vi "Main.vi"(8 "error in (no error)":errorcluster, 11 "CascadeBase in":refnum<class "Cascade.lvclass">) -> (0 "error out":errorcluster, 3 "component":refnum<class "Cascade.lvclass">)   [LabVIEW 2012, in "Cascade.lvclass"]
doc: "Main VI of the component."
uses:
  Cascade.lvclass
  <vilib>/Distrio/Murmex/Murmex/command_enum.ctl
  Cascade.lvclass/Cascade.ctl
  <vilib>/Distrio/Murmex/InitialiseMessage/InitialiseMessage.lvclass
  <vilib>/Distrio/Murmex/GenericMessage/GenericMessage.lvclass
  <vilib>/Distrio/Murmex/TerminateMessage/TerminateMessage.lvclass
  <vilib>/Distrio/Murmex/ConfigureMessage/ConfigureMessage.lvclass
  <vilib>/Distrio/Murmex/StartMessage/run mode enum.ctl
  <vilib>/Distrio/Murmex/StopMessage/StopMessage.lvclass
  <vilib>/Distrio/Murmex/StartMessage/StartMessage.lvclass
  <vilib>/Distrio/Murmex/Murmex/update_cluster.ctl
  <vilib>/Distrio/Murmex/Murmex/Murmex.lvclass
  <vilib>/Distrio/Murmex/Murmex/Set configure at initialise.vi
  <vilib>/Distrio/Murmex/Murmex/Set log reference.vi
  <vilib>/Distrio/Murmex/Murmex/Set VI reference.vi
  <vilib>/Distrio/Murmex/Murmex/Get ID.vi
  <vilib>/Distrio/Murmex/Murmex/Set write log to disk.vi
  <vilib>/Distrio/Murmex/Message/Add or replace parameter.vi
  <vilib>/Distrio/Murmex/Message/Message.lvclass
  <vilib>/vision/NI_Vision_Development_Module.lvlib
panel:
  in  "PID gains":T1
  in  "button:configure":bool
  in  "button:quit":bool
  out "terminate?":bool
  in  "Tab Control":enum32{"Settings", "Phase comparison", "Debug"}(tab)
  out "Video":T2(plugin-control)
  in  "Exposure":dbl[unit]
  in  "Gain":dbl=65535.0
  in  "button:free run":bool
  out "Status":string
  in  "Reporting folder":path=path "C:/DATA"
  in  "Filename":string="trial"
  in  "save":bool
  in  "select ROIS":bool
  out "good alignment?":bool
  out "translation":dbl[unit]
  out "pixel shift":dbl
  in  "send move":bool
  in  "AF":bool
  in  "set as focus":bool
  out "ROB":T2(plugin-control)
  out "rob":T2(plugin-control)
  out "ROY":T2(plugin-control)
  out "roy":T2(plugin-control)
  out "aligned ROIs":T2(plugin-control)
  out "log":string
  in  "Component id":string="Cascade"
  in  "button:send command":bool
  in  "generic command":string
  in  "command":T3
  in  "button:single frame":bool
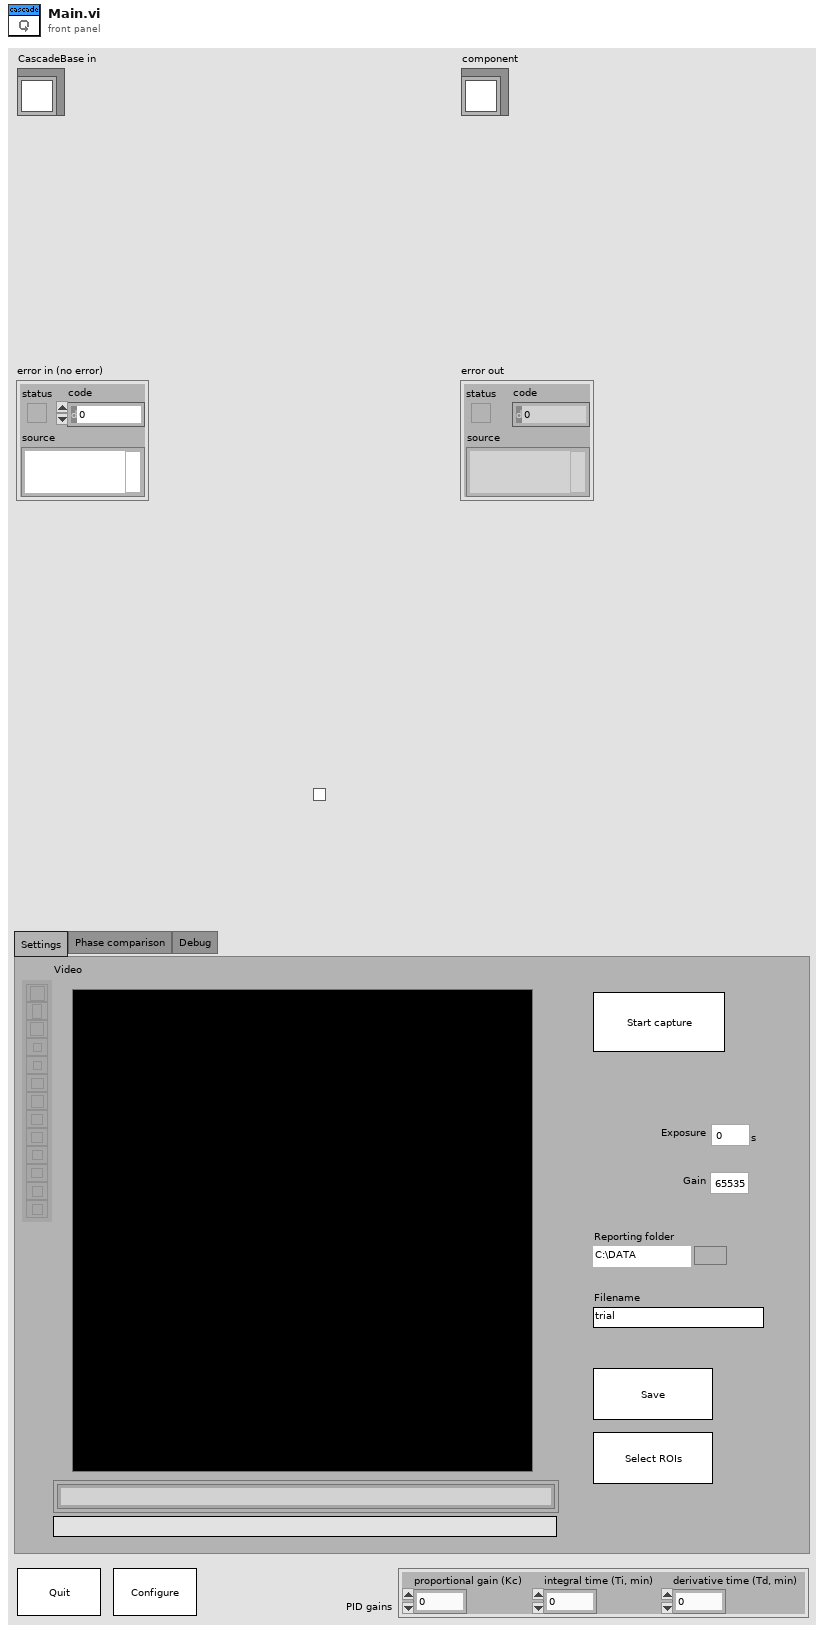
[diagram p1: front panel]
types:
  T1 = cluster{"proportional gain (Kc)":dbl, "integral time (Ti, min)":dbl, "derivative time (Td, min)":dbl}
  T2 = typedef "IMAQ Image.ctl" = refnum<image>
  T3 = typedef "Murmex.lvlib/Murmex.lvclass/command_enum.ctl" = enum16{"null", "initialise", "reset", "terminate", "acknowledge", "update", "inspect", "inform", "proceed", "start", "stop", "fetch", "configure", "generic"}
  T4 = enum8{"Enabled", "Disabled", "Disabled and Grayed Out"}
  T5 = typedef "Murmex.lvlib/StartMessage.lvclass/run mode enum.ctl" = enum16{"infinite", "finite"}
  T6 = typedef "Murmex.lvlib/Murmex.lvclass/update_cluster.ctl" = cluster{"target ID":string, "key chains":string[], "values":variant[]}
  T7 = typedef "Murmex.lvclass/command_enum.ctl" = enum16{"null", "initialise", "reset", "terminate", "acknowledge", "update", "inspect", "inform", "proceed", "start", "stop", "fetch", "configure", "generic"}
  T8 = typedef "Murmex.lvclass/Event type enumerations.ctl" = enum16{"before", "after"}
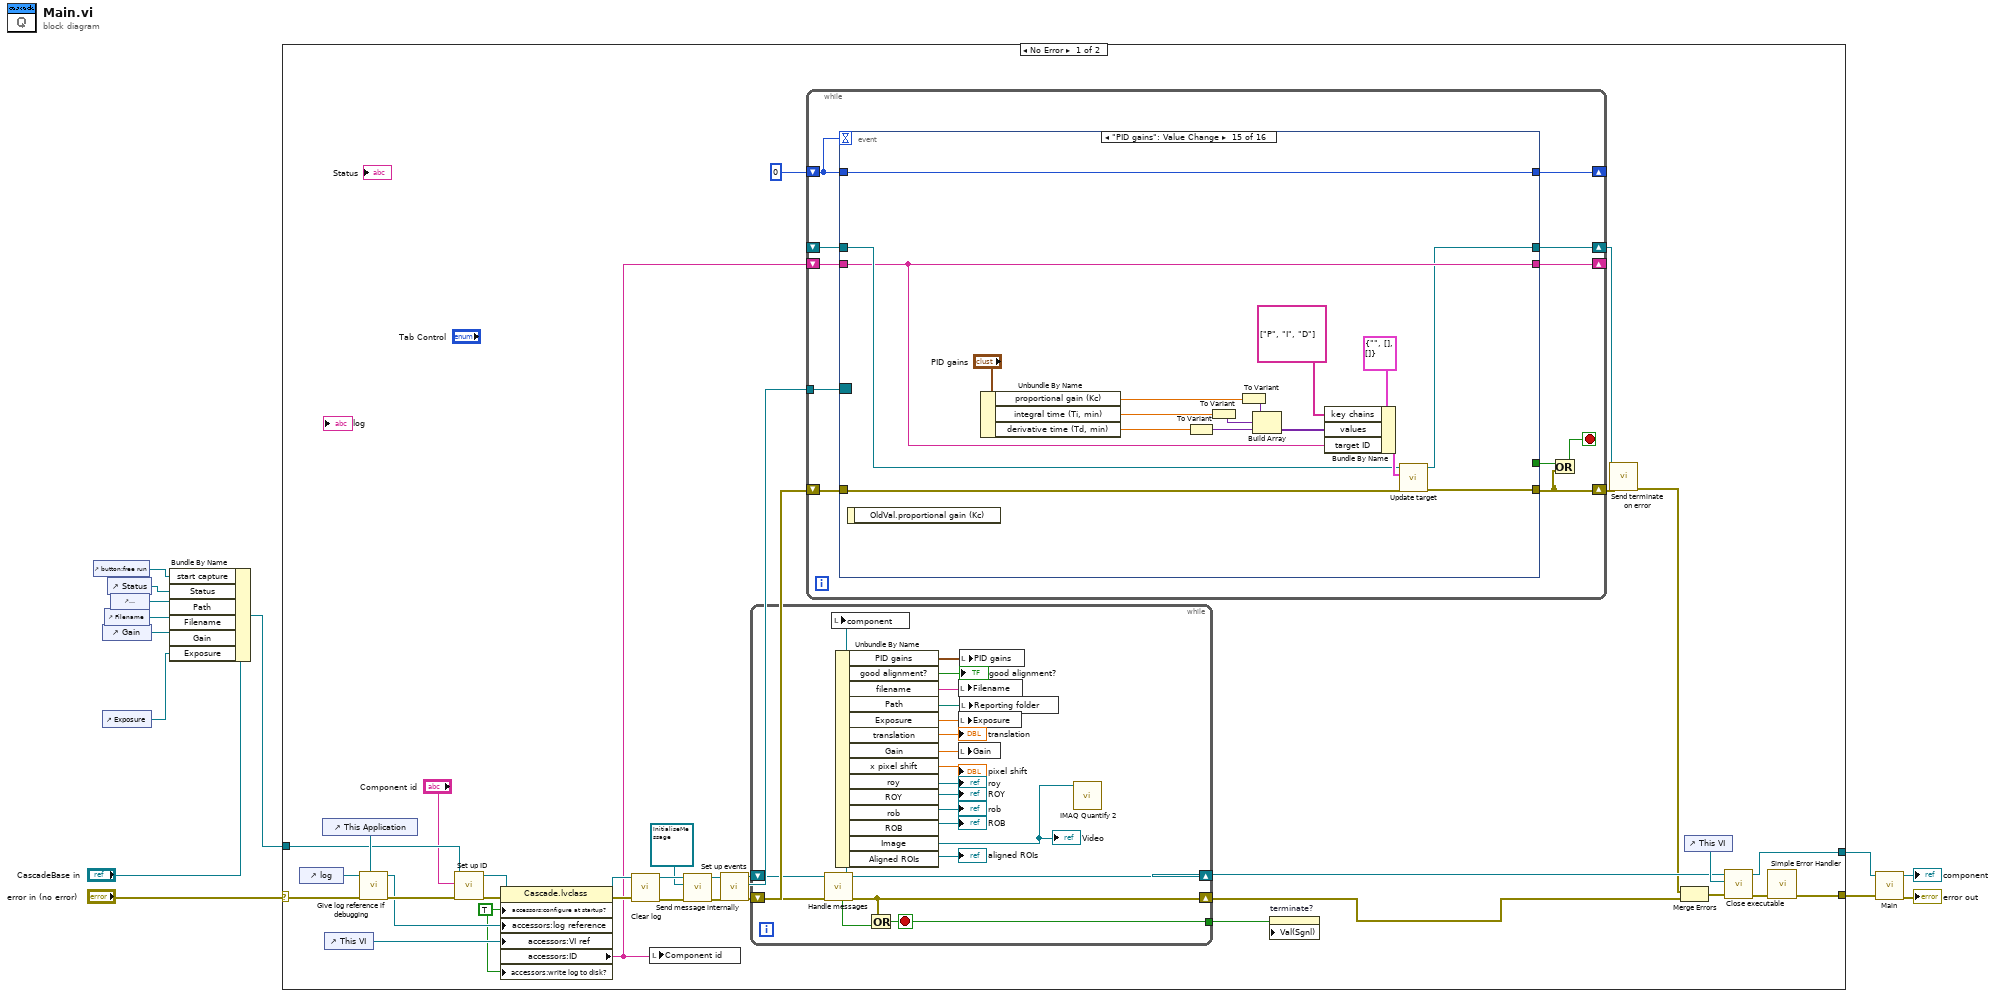
[diagram p0: block diagram]
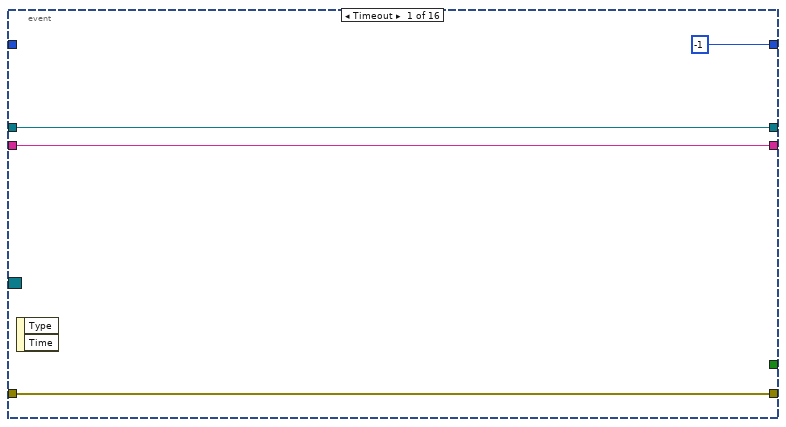
[diagram p2: hidden frame]
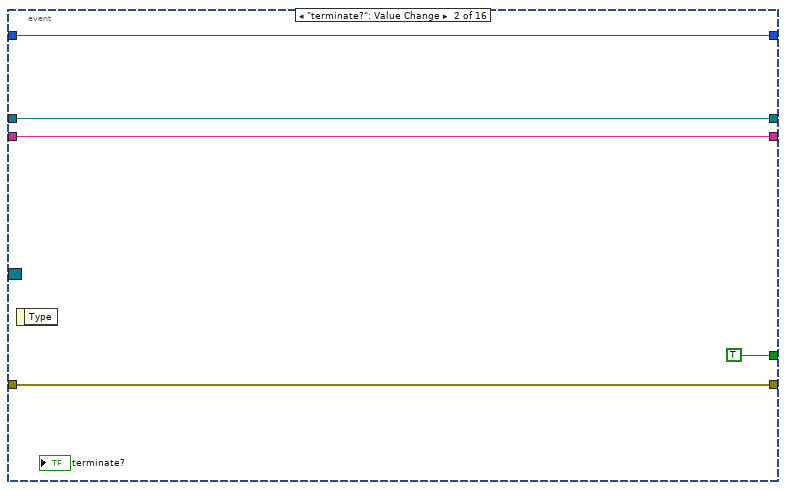
[diagram p3: hidden frame]
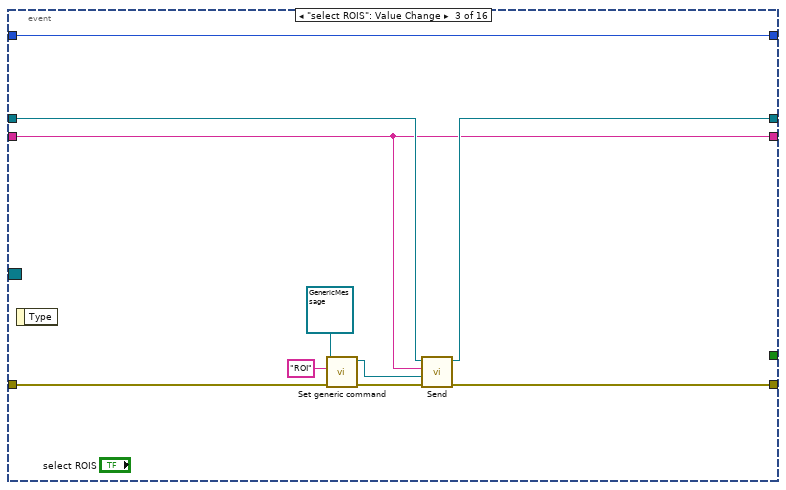
[diagram p4: hidden frame]
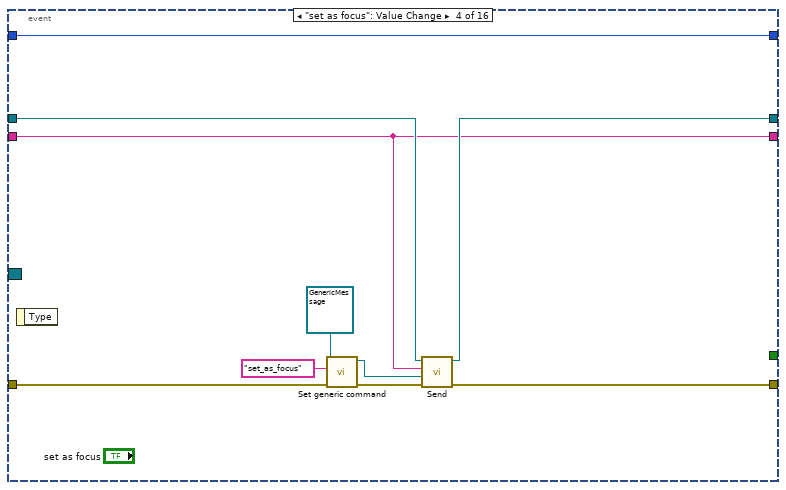
[diagram p5: hidden frame]
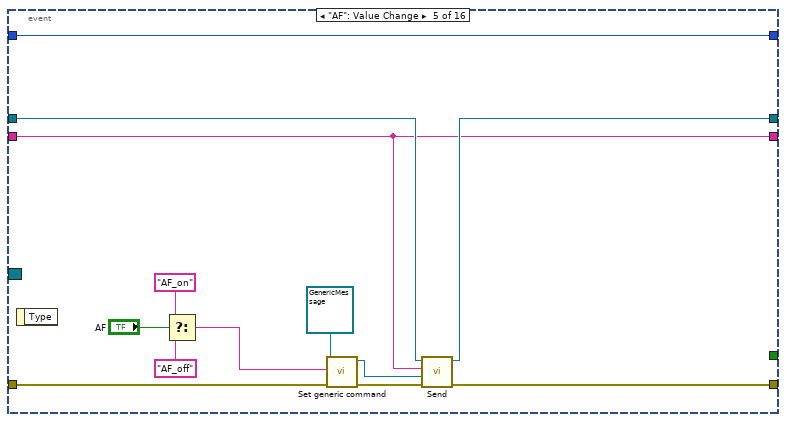
[diagram p6: hidden frame]
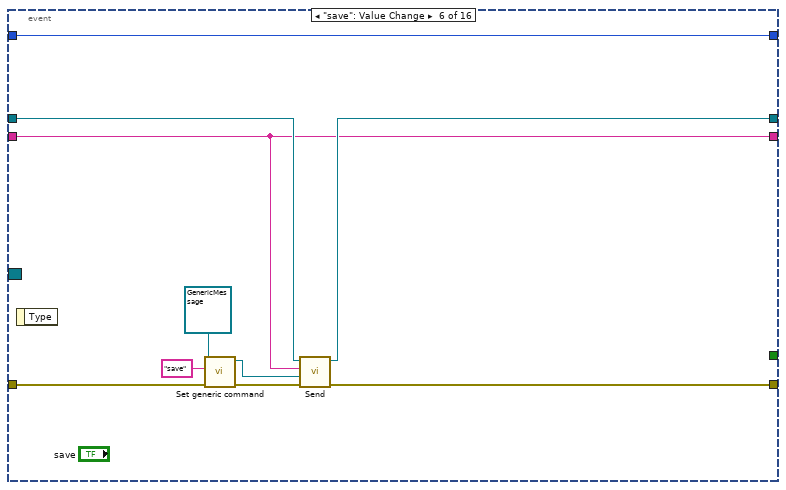
[diagram p7: hidden frame]
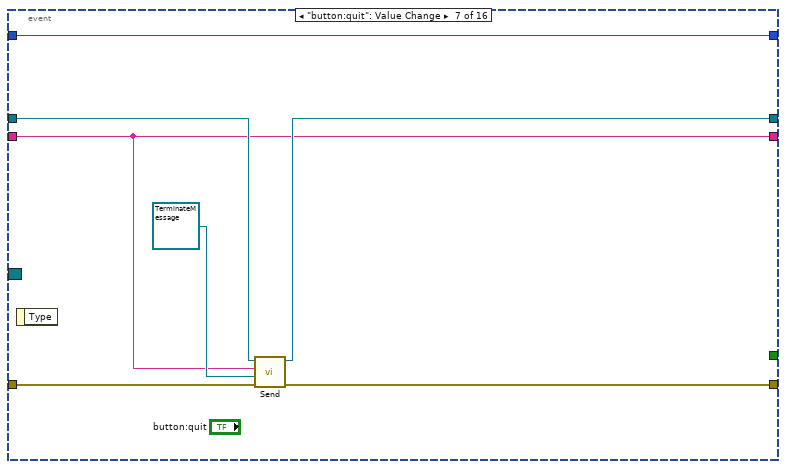
[diagram p8: hidden frame]
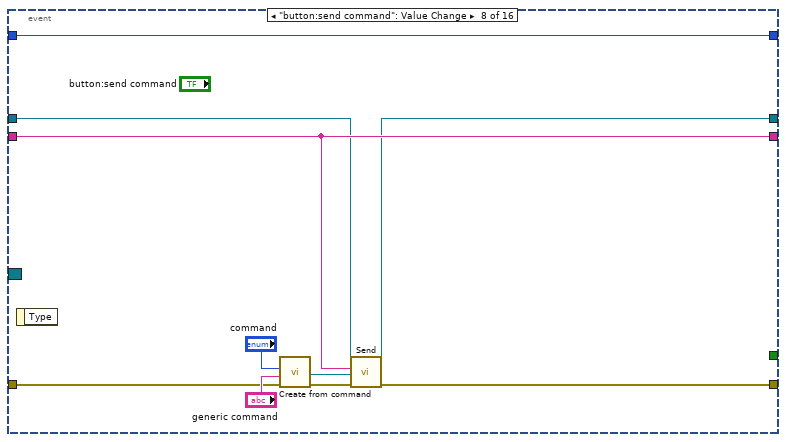
[diagram p9: hidden frame]
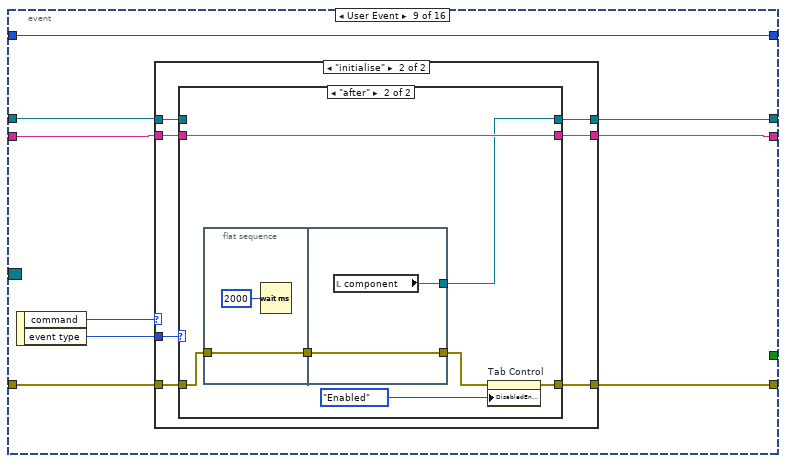
[diagram p10: hidden frame]
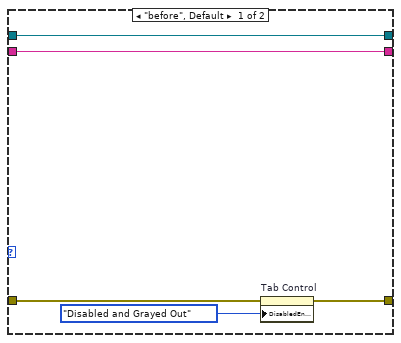
[diagram p12: hidden frame]
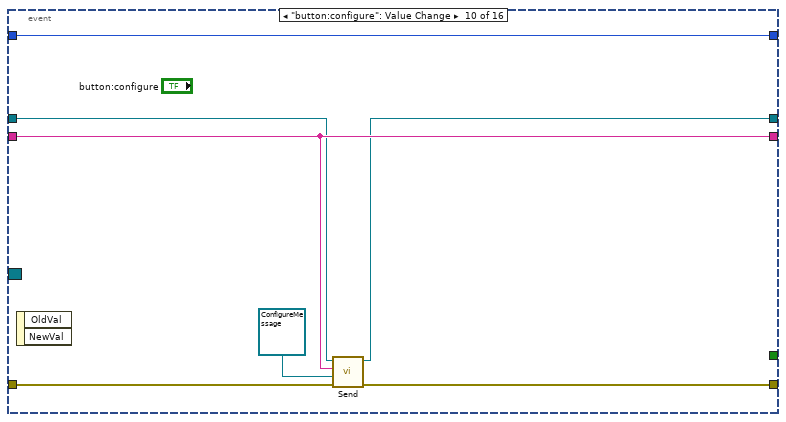
[diagram p13: hidden frame]
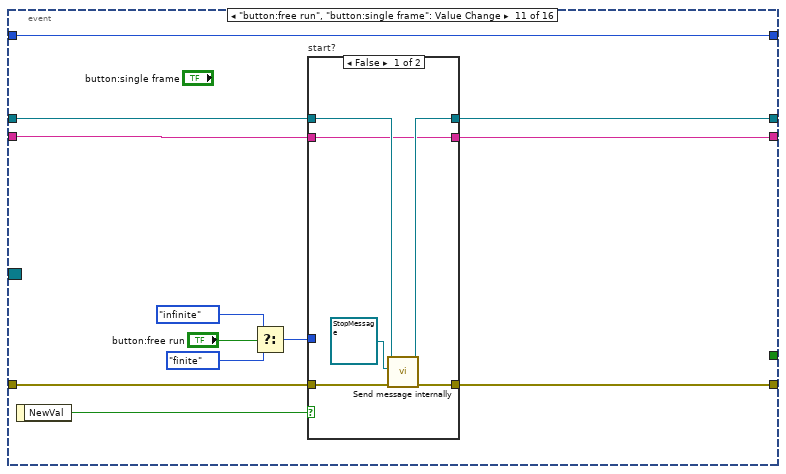
[diagram p14: hidden frame]
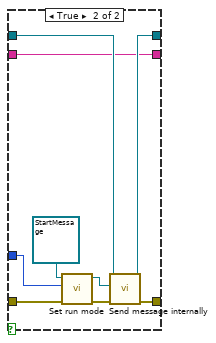
[diagram p15: hidden frame]
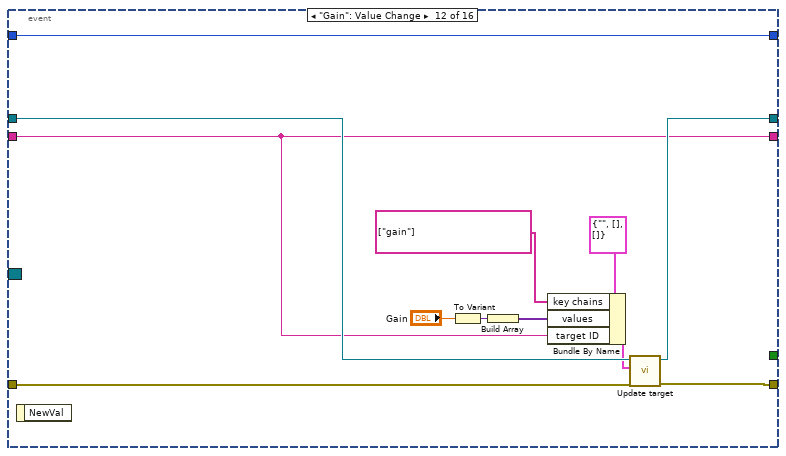
[diagram p16: hidden frame]
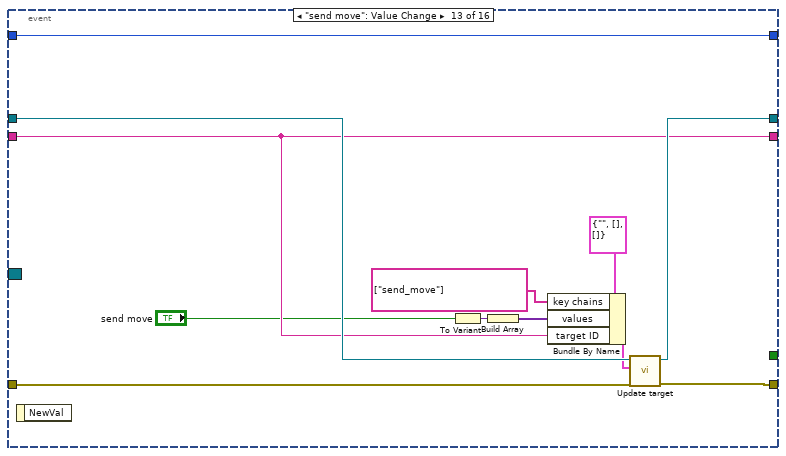
[diagram p17: hidden frame]
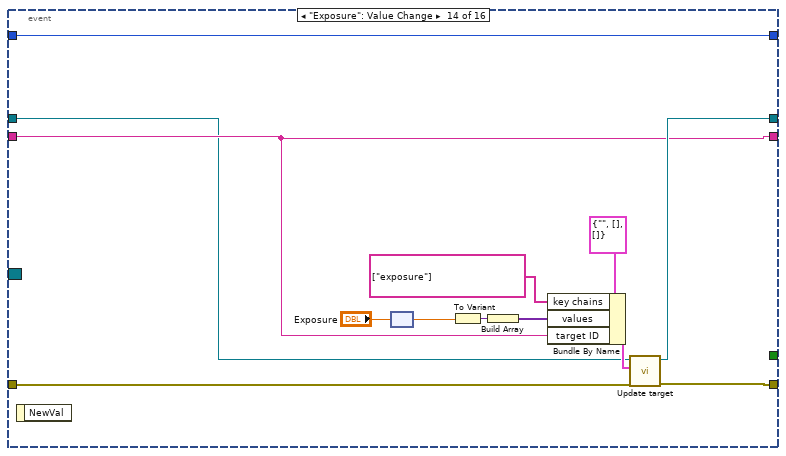
[diagram p18: hidden frame]
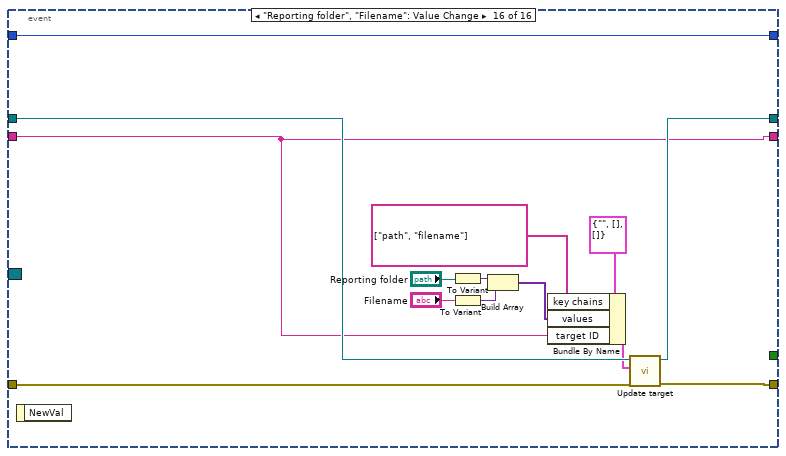
[diagram p19: hidden frame]
diagram:
  n1 = control-ref of="button:free run"() -> (w1:refnum<vi>)
  n2 = control-ref of="Gain"() -> (w5:refnum<vi>)
  n3 = control-ref of="Exposure"() -> (w6:refnum<vi>)
  n4 = control-ref of="Filename"() -> (w4:refnum<vi>)
  n5 = control-ref of="Status"() -> (w2:refnum<vi>)
  n6 = control-ref of="Reporting folder"() -> (w3:refnum<vi>)
  n7 = Bundle By Name(cluster="CascadeBase in", "start capture"=w1, "Status"=w2, "Path"=w3, "Filename"=w4, "Gain"=w5, "Exposure"=w6) -> (w10:refnum<class "Cascade.lvclass">)
  n8 = case shown="No Error" "error in (no error)" {
    selector: "error in (no error)" -> [w46 w286]
    tunnel: w10 -> [w45 w285]
    tunnel: [w19 w285] -> w9
    tunnel: [w17 w286] -> w7
    frame No Error {
      w15 = TRUE ("configure at startup?")
      n9 = control-ref of="log"() -> (w39:refnum<vi>)
      n10 = control-ref of="This Application"() -> (w47:refnum<vi>)
      n11 = control-ref of="This VI"() -> (w38:refnum<vi>)
      n12 = call "Give log reference if debugging.vi"("application ref"=w47, "error in (no error)"=w46, "log reference in"=w39) -> ("error out"=w44:errorcluster, "log reference out"=w40:refnum<vi>)  [unwired: 6 in, 1 out]
      n13 = call <vilib>:"Set up ID.vi"("error in (no error)"=w44, "component ID"="Component id", "MurmexBase in"=w45) -> ("error out"=w42:errorcluster, "MurmexBase out"=w41:refnum<class "Cascade.lvclass">)  [unwired: 6 in, 1 out]
      n14 = property class="Cascade.lvclass"(reference=w41, error in=w42, "accessors:configure at startup?"=w15, "accessors:log reference"=w40, "accessors:VI ref"=w38, "accessors:write log to disk?"=w15) -> (reference out=w31:refnum<class "Cascade.lvclass">, error out=w33:errorcluster, "accessors:ID"=w27:string)
      n15 = call <vilib>:"Clear log.vi"("error in (no error)"=w33, "MurmexBase in"=w31) -> ("error out"=w36:errorcluster, "MurmexBase out"=w37:refnum<class "Cascade.lvclass">)  [unwired: 8 in]
      n16 = local write "Component id"(w27) -> ()
      n17 = call <vilib>:"Send message internally.vi"("error in (no error)"=w36, "Message"=refnum<class "InitialiseMessage.lvclass"> refnum ("InitialiseMessage"), "Murmex in"=w37) -> ("error out"=w35:errorcluster, "Murmex out"=w34:refnum<class "Cascade.lvclass">)  [unwired: 7 in]
      n18 = call <vilib>:"Set up events.vi"("error in (no error)"=w35, "MurmexBase in"=w34) -> ("error out"=w28:errorcluster, "Event Registration Refnum"=w30:refnum<event-registration>, "MurmexBase out"=w29:refnum<class "Cascade.lvclass">)  [unwired: 7 in]
      n19 = while {
        shift-right: [w282] -> w14
        shift-left: w28 -> [w284]
        shift-right: [w279] -> w20
        shift-left: w29 -> [w280]
        tunnel: [w281] -> w16
        stop <- w281 stop-if-true
        n20 = call <vilib>:"Handle messages.vi"("error in (no error)"=w284, "Murmex in"=w280) -> ("error out"=w282:errorcluster, "Murmex out"=w279:refnum<class "Cascade.lvclass">, "terminated?"=w283:bool)  [unwired: 7 in]
        n21 = local write "component"(w279) -> ()
        n22 = Unbundle By Name(w279) -> ("PID gains"=w265:T1, "good alignment?"=→"good alignment?":bool, "filename"=w268:string, "Path"=w267:path, "Exposure"=w269:dbl[unit], "translation"=→"translation":dbl[unit], "Gain"=w270:dbl, "x pixel shift"=→"pixel shift":dbl, "roy"=→"roy":T2, "ROY"=→"ROY":T2, "rob"=→"rob":T2, "ROB"=→"ROB":T2, "Image"=w271:T2, "Aligned ROIs"=→"aligned ROIs":T2)
        "Video" <- w271
        n23 = Or(x=w282, y=w283) -> (x .or. y?=w281:bool)
        n24 = local write "Filename"(w268) -> ()
        n25 = local write "Exposure"(w269) -> ()
        n26 = local write "Gain"(w270) -> ()
        n27 = local write "PID gains"(w265) -> ()
        n28 = local write "Reporting folder"(w267) -> ()
        n29 = call "IMAQ Quantify 2"("Image"=w271) -> ()  [unwired: 8 in, 3 out]
      }
      n30 = while {
        tunnel: w30 -> [w58]
        shift-right: [w50] -> w25
        shift-left: w28 -> [w57]
        shift-right: [w55] -> _
        shift-left: 0 -> [w54]
        shift-right: [w53] -> _
        shift-left: w27 -> [w56]
        shift-right: [w52] -> w24
        shift-left: _ -> [w51]
        stop <- w49 stop-if-true
        n31 = event shown="[14] \"PID gains\": Value Change" {
          selector: w58 -> [_ _ _ _ _ _ _ _ _ _ _ _ _ _ _ _]
          dyn-events: _ -> [_ _ _ _ _ _ _ _ _ _ _ _ _ _ _ _]
          timeout: w54 -> [_ _ _ _ _ _ _ _ _ _ _ _ _ _ _ _]
          tunnel: w57 -> [w61 w66 w73 w83 w97 w105 w117 w123 w136 w167 w180 w207 w219 w232 w243 w263]
          tunnel: w56 -> [w60 w65 w70 w80 w94 w101 w112 w121 w132 w165 w173 w197 w210 w223 w244 w254]
          tunnel: w54 -> [_ w63 w68 w78 w92 w110 w111 w118 w128 w169 w181 w199 w211 w225 w240 w255]
          tunnel: [-1 w63 w68 w78 w92 w110 w111 w118 w128 w169 w181 w199 w211 w225 w240 w255] -> w55
          tunnel: [w61 w66 w69 w79 w93 w104 w116 w122 w135 w166 w179 w208 w220 w233 w242 w264] -> w50
          tunnel: [w60 w65 w70 w80 w94 w101 w112 w121 w131 w165 w170 w197 w210 w223 w244 w254] -> w53
          tunnel: [w59 w64 w71 w81 w95 w102 w113 w119 w130 w163 w171 w206 w218 w231 w241 w262] -> w52
          tunnel: w51 -> [w59 w64 w72 w82 w96 w103 w114 w120 w129 w164 w172 w205 w217 w221 w245 w261]
          tunnel: [_ TRUE _ _ _ _ _ _ _ _ _ _ _ _ _ _] -> w48
          event Timeout {
            n32 = event-data() -> ()  [unwired: 1 in, 2 out]
          }
          event "terminate?": Value Change {
            n33 = event-data() -> ()  [unwired: 1 in, 1 out]
          }
          event "select ROIS": Value Change {
            n34 = event-data() -> ()  [unwired: 1 in, 1 out]
            n35 = call <vilib>:"Set generic command.vi"("error in (no error)"=w73, "generic command"="ROI", "GenericMessage in"=refnum<class "GenericMessage.lvclass"> refnum ("Message in")) -> ("error out"=w74:errorcluster, "GenericMessage out"=w76:refnum<class "GenericMessage.lvclass">)  [unwired: 7 in]
            n36 = call <vilib>:"Send.vi"("error in (no error)"=w74, "Message"=w76, "recipient"=w70, "Murmex in"=w72) -> ("error out"=w69:errorcluster, "Murmex out"=w71:refnum<class "Murmex.lvclass">)  [unwired: 6 in]
          }
          event "set as focus": Value Change {
            n37 = event-data() -> ()  [unwired: 1 in, 1 out]
            n38 = call <vilib>:"Set generic command.vi"("error in (no error)"=w83, "generic command"="set_as_focus", "GenericMessage in"=refnum<class "GenericMessage.lvclass"> refnum ("Message in")) -> ("error out"=w84:errorcluster, "GenericMessage out"=w86:refnum<class "GenericMessage.lvclass">)  [unwired: 7 in]
            n39 = call <vilib>:"Send.vi"("error in (no error)"=w84, "Message"=w86, "recipient"=w80, "Murmex in"=w82) -> ("error out"=w79:errorcluster, "Murmex out"=w81:refnum<class "Murmex.lvclass">)  [unwired: 6 in]
          }
          event "AF": Value Change {
            n40 = event-data() -> ()  [unwired: 1 in, 1 out]
            n41 = Select(t="AF_on" ("generic command"), s="AF", f="AF_off" ("generic command")) -> (s? t:f=w88:string)
            n42 = call <vilib>:"Set generic command.vi"("error in (no error)"=w97, "generic command"=w88, "GenericMessage in"=refnum<class "GenericMessage.lvclass"> refnum ("Message in")) -> ("error out"=w98:errorcluster, "GenericMessage out"=w100:refnum<class "GenericMessage.lvclass">)  [unwired: 7 in]
            n43 = call <vilib>:"Send.vi"("error in (no error)"=w98, "Message"=w100, "recipient"=w94, "Murmex in"=w96) -> ("error out"=w93:errorcluster, "Murmex out"=w95:refnum<class "Murmex.lvclass">)  [unwired: 6 in]
          }
          event "save": Value Change {
            n44 = event-data() -> ()  [unwired: 1 in, 1 out]
            n45 = call <vilib>:"Set generic command.vi"("error in (no error)"=w105, "generic command"="save", "GenericMessage in"=refnum<class "GenericMessage.lvclass"> refnum ("Message in")) -> ("error out"=w106:errorcluster, "GenericMessage out"=w108:refnum<class "GenericMessage.lvclass">)  [unwired: 7 in]
            n46 = call <vilib>:"Send.vi"("error in (no error)"=w106, "Message"=w108, "recipient"=w101, "Murmex in"=w103) -> ("error out"=w104:errorcluster, "Murmex out"=w102:refnum<class "Murmex.lvclass">)  [unwired: 6 in]
          }
          event "button:quit": Value Change {
            n47 = event-data() -> ()  [unwired: 1 in, 1 out]
            n48 = call <vilib>:"Send.vi"("error in (no error)"=w117, "Message"=refnum<class "TerminateMessage.lvclass"> refnum ("TerminateMessage"), "recipient"=w112, "Murmex in"=w114) -> ("error out"=w116:errorcluster, "Murmex out"=w113:refnum<class "Murmex.lvclass">)  [unwired: 6 in]
          }
          event "button:send command": Value Change {
            n49 = event-data() -> ()  [unwired: 1 in, 1 out]
            n50 = call <vilib>:"Create from command.vi"("error in (no error)"=w123, "generic command"="generic command", "command"="command") -> ("error out"=w124:errorcluster, "Message out"=w127:refnum<class "Message.lvclass">)  [unwired: 7 in]
            n51 = call <vilib>:"Send.vi"("error in (no error)"=w124, "Message"=w127, "recipient"=w121, "Murmex in"=w120) -> ("error out"=w122:errorcluster, "Murmex out"=w119:refnum<class "Murmex.lvclass">)  [unwired: 6 in]
          }
          event User Event {
            n52 = event-data() -> ("command"=w133:T7, "event type"=w134:T8)  [unwired: 1 in]
            n53 = case shown="\"initialise\"" w133 {
              tunnel: w134 -> [_ w146]
              tunnel: w136 -> [w137 w145]
              tunnel: w132 -> [w138 w144]
              tunnel: [w138 w143] -> w131
              tunnel: [w139 w142] -> w130
              tunnel: w129 -> [w139 w141]
              tunnel: [w137 w140] -> w135
              frame "null", Default {
              }
              frame "initialise" {
                n54 = case shown="\"after\"" w146 {
                  tunnel: w145 -> [w148 w153]
                  tunnel: [w147 w157] -> w140
                  tunnel: [w150 w156] -> w143
                  tunnel: w144 -> [w150 w156]
                  tunnel: [w151 w155] -> w142
                  tunnel: w141 -> [w151 _]
                  frame "before", Default {
                    n55 = property on="Tab Control" class="TabCtl (strict)"(error in=w148, "DisabledEnum"=T4."Disabled and Grayed Out" ("Disabled")) -> (error out=w147:errorcluster)  [unwired: 1 in, 1 out]
                  }
                  frame "after" {
                    n56 = flat-sequence {
                      tunnel: [w160] -> w154
                      tunnel: w153 -> [w160]
                      tunnel: [w162] -> w155
                      tunnel: [w161] -> w152
                      tunnel: w154 -> [w161]
                      frame #0 {
                        n57 = Wait (ms)(milliseconds to wait=u32 2000) -> ()  [unwired: 1 out]
                      }
                      frame #1 {
                        n58 = local read "component"() -> (w162:refnum<class "Cascade.lvclass">)
                      }
                    }
                    n59 = property on="Tab Control" class="TabCtl (strict)"(error in=w152, "DisabledEnum"=T4."Enabled" ("Disabled")) -> (error out=w157:errorcluster)  [unwired: 1 in, 1 out]
                  }
                }
              }
            }
          }
          event "button:configure": Value Change {
            n60 = event-data() -> ()  [unwired: 1 in, 2 out]
            n61 = call <vilib>:"Send.vi"("error in (no error)"=w167, "Message"=refnum<class "ConfigureMessage.lvclass"> refnum ("ConfigureMessage"), "recipient"=w165, "Murmex in"=w164) -> ("error out"=w166:errorcluster, "Murmex out"=w163:refnum<class "Murmex.lvclass">)  [unwired: 6 in]
          }
          event "button:free run", "button:single frame": Value Change {
            n62 = event-data() -> ("NewVal"=w178:bool)  [unwired: 1 in]
            n63 = Select(t=run_mode_enum."infinite" ("run mode"), s="button:free run", f=run_mode_enum."finite" ("run mode")) -> (s? t:f=w174:T5)
            n64 = case "start?" shown="False" w178 {
              tunnel: w180 -> [w187 w191]
              tunnel: [w186 w194] -> w179
              tunnel: w172 -> [w185 w196]
              tunnel: [w184 w195] -> w171
              tunnel: w173 -> [w183 w193]
              tunnel: [w183 w193] -> w170
              tunnel: w174 -> [_ w192]
              frame False {
                n65 = call <vilib>:"Send message internally.vi"("error in (no error)"=w187, "Message"=refnum<class "StopMessage.lvclass"> refnum ("Distrio Murmex 1.5:StopMessage"), "Murmex in"=w185) -> ("error out"=w186:errorcluster, "Murmex out"=w184:refnum<class "Murmex.lvclass">)  [unwired: 7 in]
              }
              frame True {
                n66 = call <vilib>:"Set run mode.vi"("error in (no error)"=w191, "run mode"=w192, "StartMessage in"=refnum<class "StartMessage.lvclass"> refnum ("Message in")) -> ("error out"=w190:errorcluster, "StartMessage out"=w188:refnum<class "StartMessage.lvclass">)  [unwired: 7 in]
                n67 = call <vilib>:"Send message internally.vi"("error in (no error)"=w190, "Message"=w188, "Murmex in"=w196) -> ("error out"=w194:errorcluster, "Murmex out"=w195:refnum<class "Murmex.lvclass">)  [unwired: 7 in]
              }
            }
          }
          event "Gain": Value Change {
            n68 = event-data() -> ()  [unwired: 1 in, 1 out]
            n69 = To Variant(anything="Gain") -> (Variant=w203:variant)
            n70 = Build Array(w203) -> (w204:variant[])
            n71 = Bundle By Name(cluster=T6 {"target ID"="", "key chains"=[], "values"=[]} ("update cluster"), "key chains"=string[] ["gain"], "values"=w204, "target ID"=w197) -> (w201:T6)
            n72 = call <vilib>:"Update target.vi"("error in (no error)"=w207, "update cluster"=w201, "MurmexBase in"=w205) -> ("error out"=w208:errorcluster, "MurmexBase out"=w206:refnum<class "Murmex.lvclass">)  [unwired: 7 in]
          }
          event "send move": Value Change {
            n73 = event-data() -> ()  [unwired: 1 in, 1 out]
            n74 = To Variant(anything="send move") -> (Variant=w215:variant)
            n75 = Build Array(w215) -> (w216:variant[])
            n76 = Bundle By Name(cluster=T6 {"target ID"="", "key chains"=[], "values"=[]} ("update cluster"), "key chains"=string[] ["send_move"], "values"=w216, "target ID"=w210) -> (w213:T6)
            n77 = call <vilib>:"Update target.vi"("error in (no error)"=w219, "update cluster"=w213, "MurmexBase in"=w217) -> ("error out"=w220:errorcluster, "MurmexBase out"=w218:refnum<class "Murmex.lvclass">)  [unwired: 7 in]
          }
          event "Exposure": Value Change {
            n78 = event-data() -> ()  [unwired: 1 in, 1 out]
            n79 = node("Exposure") -> (w222:dbl)
            n80 = To Variant(anything=w222) -> (Variant=w229:variant)
            n81 = Build Array(w229) -> (w230:variant[])
            n82 = Bundle By Name(cluster=T6 {"target ID"="", "key chains"=[], "values"=[]} ("update cluster"), "key chains"=string[] ["exposure"], "values"=w230, "target ID"=w223) -> (w227:T6)
            n83 = call <vilib>:"Update target.vi"("error in (no error)"=w232, "update cluster"=w227, "MurmexBase in"=w221) -> ("error out"=w233:errorcluster, "MurmexBase out"=w231:refnum<class "Murmex.lvclass">)  [unwired: 7 in]
          }
          event "PID gains": Value Change {
            n84 = event-data() -> ()  [unwired: 1 in, 1 out]
            n85 = Unbundle By Name("PID gains") -> ("proportional gain (Kc)"=w238:dbl, "integral time (Ti, min)"=w237:dbl, "derivative time (Td, min)"=w236:dbl)
            n86 = To Variant(anything=w236) -> (Variant=w249:variant)
            n87 = To Variant(anything=w237) -> (Variant=w235:variant)
            n88 = To Variant(anything=w238) -> (Variant=w234:variant)
            n89 = Build Array(w234, w235, w249) -> (w250:variant[])
            n90 = Bundle By Name(cluster=T6 {"target ID"="", "key chains"=[], "values"=[]} ("update cluster"), "key chains"=string[] ["P", "I", "D"], "values"=w250, "target ID"=w244) -> (w247:T6)
            n91 = call <vilib>:"Update target.vi"("error in (no error)"=w243, "update cluster"=w247, "MurmexBase in"=w245) -> ("error out"=w242:errorcluster, "MurmexBase out"=w241:refnum<class "Murmex.lvclass">)  [unwired: 7 in]
          }
          event "Reporting folder", "Filename": Value Change {
            n92 = event-data() -> ()  [unwired: 1 in, 1 out]
            n93 = To Variant(anything="Reporting folder") -> (Variant=w259:variant)
            n94 = To Variant(anything="Filename") -> (Variant=w251:variant)
            n95 = Build Array(w259, w251) -> (w260:variant[])
            n96 = Bundle By Name(cluster=T6 {"target ID"="", "key chains"=[], "values"=[]} ("update cluster"), "key chains"=string[] ["path", "filename"], "values"=w260, "target ID"=w254) -> (w257:T6)
            n97 = call <vilib>:"Update target.vi"("error in (no error)"=w263, "update cluster"=w257, "MurmexBase in"=w261) -> ("error out"=w264:errorcluster, "MurmexBase out"=w262:refnum<class "Murmex.lvclass">)  [unwired: 7 in]
          }
        }
        n98 = Or(x=w48, y=w50) -> (x .or. y?=w49:bool)
      }
      n99 = property on="terminate?" class="Bool (strict)"("Val(Sgnl)"=w16) -> ()  [unwired: 2 in, 2 out]
      n100 = call <vilib>:"Send terminate on error.vi"("error in (no error)"=w25, "Murmex in"=w24) -> ("error out"=w18:errorcluster)  [unwired: 8 in, 1 out]
      n101 = Merge Errors(w18, w14) -> (w22:errorcluster)
      n102 = control-ref of="This VI"() -> (w21:refnum<vi>)
      n103 = call <vilib>:"Close executable.vi"("error in (no error)"=w22, "main VI ref (optional)"=w21, "MurmexBase in"=w20) -> ("error out"=w23:errorcluster, "MurmexBase out"=w19:refnum<class "Cascade.lvclass">)  [unwired: 7 in]
      n104 = call <vilib>:"Simple Error Handler.vi"("error in (no error)"=w23) -> ("error out"=w17:errorcluster)  [unwired: 4 in, 4 out]
    }
    frame Error {
    }
  }
  n105 = call-parent "Main.vi"("error in (no error)"=w7, "Murmex in"=w9) -> ("error out"=→"error out":errorcluster, "Murmex out"=→"component":refnum<class "Cascade.lvclass">)  [unwired: 8 in]
